vi "InitiateAxis.vi"(0 "Axis in":refnum<class "Axis.lvclass">, 1 "m_Node":refnum<k24>, 2 "m_sysMgr":refnum<k24>, 3 "error in (no error)":errorcluster) -> (7 "Axis out":refnum<class "Axis.lvclass">, 10 "error out":errorcluster)   [LabVIEW 2020, in "Axis.lvclass"]
uses:
  Axis.lvclass
  C:/Users/Jonathan/Documents/Clearpath SDK/CSharp Examples/CLRWrapper/x64/Debug/CLRWrapper.dll
  CSharp Examples/CLRWrapper/x64/Debug/CLRWrapper.dll
  Axis.lvclass/Axis.ctl
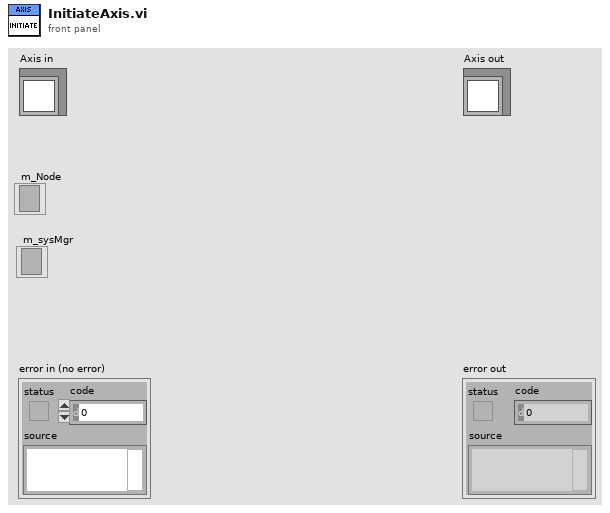
[diagram p1: front panel]
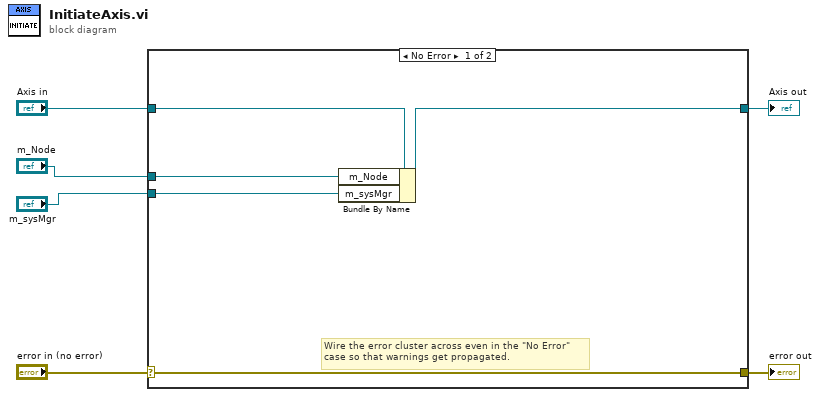
[diagram p0: block diagram]
diagram:
  n1 = case shown="No Error" "error in (no error)" {
    selector: "error in (no error)" -> [w11 w13]
    tunnel: [w11 w13] -> w5
    tunnel: [w10 w12] -> w3
    tunnel: "Axis in" -> [w9 w12]
    tunnel: "m_sysMgr" -> [w8 _]
    tunnel: "m_Node" -> [w7 _]
    frame No Error {
      # "Wire the error cluster across even in the \"No Error\"\ncase so that warnings get propagated."
      n2 = Bundle By Name(cluster=w9, "m_Node"=w7, "m_sysMgr"=w8) -> (w10:refnum<class "Axis.lvclass">)
    }
    frame Error {
    }
  }
  "error out" <- w5
  "Axis out" <- w3
